vi "Lat-Long Deg to M-S.vi"(9 "Long Deg":dbl=-122.2170661, 11 "Lat Deg":dbl=47.4828776) -> (1 "Long Min-Sec":string="12214.0164,W", 3 "Lat Min-Sec":string="4728.3818,N")   [LabVIEW 2024, in "EQMF.lvlib" / "Math Utils.lvlib"]
uses:
  Math Utils.lvlib
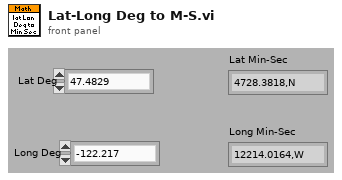
[diagram p1: front panel]
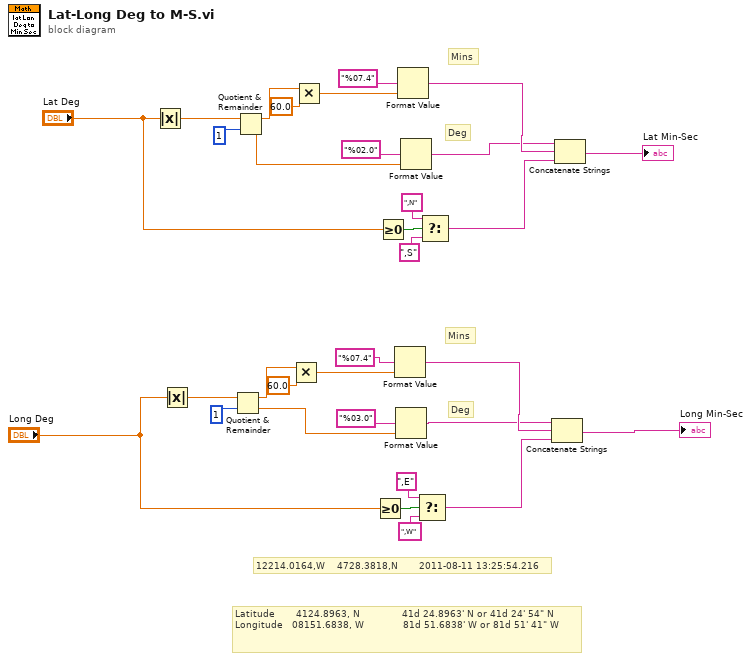
[diagram p0: block diagram]
diagram:
  # "Mins"
  # "Deg"
  # "Mins"
  # "Deg"
  # "12214.0164,W    4728.3818,N       2011-08-11 13:25:54.216"
  # "Latitude       4124.8963, N              41d 24.8963' N or 41d 24' 54\" N \nLongitude   08151.6838, W             81d 51.6838' W or 81d 51' 41\" W"
  n1 = Absolute Value(x="Lat Deg") -> (abs(x)=w9:dbl)
  n2 = Absolute Value(x="Long Deg") -> (abs(x)=w8:dbl)
  n3 = Quotient & Remainder(x=w8, y=1) -> (x-y*floor(x/y)=w14:dbl, floor(x/y)=w2:dbl)
  n4 = Quotient & Remainder(x=w9, y=1) -> (x-y*floor(x/y)=w31:dbl, floor(x/y)=w3:dbl)
  n5 = Multiply(x=w14, y=60.0) -> (x*y=w20:dbl)
  n6 = Multiply(x=w31, y=60.0) -> (x*y=w26:dbl)
  n7 = Greater Or Equal To 0?(x="Long Deg") -> (x >= 0?=w17:bool)
  n8 = Greater Or Equal To 0?(x="Lat Deg") -> (x >= 0?=w28:bool)
  n9 = Format Value(format string="%07.4", value (0)=w20) -> (output string=w21:string)  [unwired: 1 in]
  n10 = Format Value(format string="%03.0", value (0)=w2) -> (output string=w1:string)  [unwired: 1 in]
  n11 = Format Value(format string="%07.4", value (0)=w26) -> (output string=w25:string)  [unwired: 1 in]
  n12 = Format Value(format string="%02.0", value (0)=w3) -> (output string=w4:string)  [unwired: 1 in]
  n13 = Select(t=",E", s=w17, f=",W") -> (s? t:f=w22:string)
  n14 = Select(t=",N", s=w28, f=",S") -> (s? t:f=w24:string)
  n15 = Concatenate Strings(w1, w21, w22) -> (→"Long Min-Sec":string)
  n16 = Concatenate Strings(w4, w25, w24) -> (→"Lat Min-Sec":string)
